vi "getdate.vi"() -> (0 "date/time string":string)   [LabVIEW 2013]
panel:
  in  "hour cutoff":i32=7
  out "hour":string
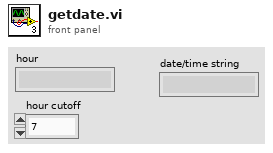
[diagram p1: front panel]
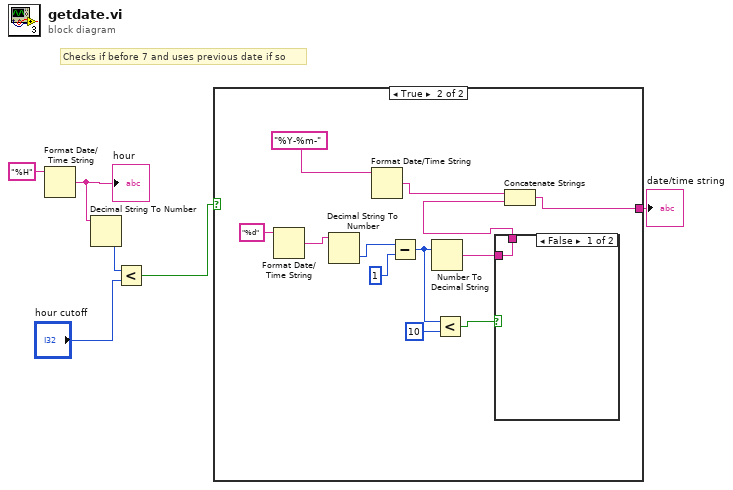
[diagram p0: block diagram]
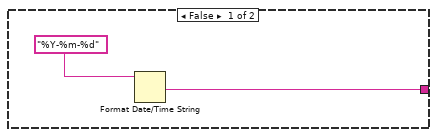
[diagram p2: hidden frame]
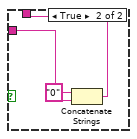
[diagram p3: hidden frame]
diagram:
  # "Checks if before 7 and uses previous date if so"
  n1 = Format Date/Time String(time format string (%c)="%H") -> (date/time string=w2:string)  [unwired: 2 in]
  "hour" <- w2
  n2 = Decimal String To Number(string=w2) -> (number=w1:i32)  [unwired: 2 in, 1 out]
  n3 = Less?(x=w1, y="hour cutoff") -> (x < y?=w4:bool)
  n4 = case shown="True" w4 {
    tunnel: [w7 w14] -> w3
    frame False {
      n5 = Format Date/Time String(time format string (%c)="%Y-%m-%d") -> (date/time string=w7:string)  [unwired: 2 in]
    }
    frame True {
      n6 = Format Date/Time String(time format string (%c)="%d") -> (date/time string=w18:string)  [unwired: 2 in]
      n7 = Decimal String To Number(string=w18) -> (number=w17:i32)  [unwired: 2 in, 1 out]
      n8 = Format Date/Time String(time format string (%c)="%Y-%m-") -> (date/time string=w15:string)  [unwired: 2 in]
      n9 = Subtract(x=w17, y=1) -> (x-y=w12:i32)
      n10 = Number To Decimal String(number=w12) -> (decimal integer string=w13:string)  [unwired: 1 in]
      n11 = Less?(x=w12, y=10) -> (x < y?=w10:bool)
      n12 = case shown="False" w10 {
        tunnel: w13 -> [w21 w24]
        tunnel: [w21 w22] -> w9
        frame False {
        }
        frame True {
          n13 = Concatenate Strings("0" ("string"), w24) -> (w22:string)
        }
      }
      n14 = Concatenate Strings(w15, w9) -> (w14:string)
    }
  }
  "date/time string" <- w3
